vi "Read Timestamp Configuration.vi"(8 "error in (no error)":errorcluster, 9 "Default If Not Found":timestamp, 10 "Name":string, 11 "database-configuration in":refnum<class "configuration-database.lvclass">) -> (0 "error out":errorcluster, 1 "Not Found?":bool, 2 "Value":timestamp, 3 "database-configuration out":refnum<class "configuration-database.lvclass">)   [LabVIEW 2020, in "configuration-database.lvlib" / "configuration-database.lvclass"]
uses:
  configuration-database.lvclass
  configuration-database.lvclass/configuration-database.ctl
  bcf94244-2e74-4bc5-bce3-b07433e8a1bf.vi
  <vilib>/Utility/error.llb/Error Cluster From Error Code.vi
  IConfigDBQueries/IConfigurationDatabaseQueries.lvclass
  externals/database-interface/IDatabase/IDatabase/IDatabase.lvclass
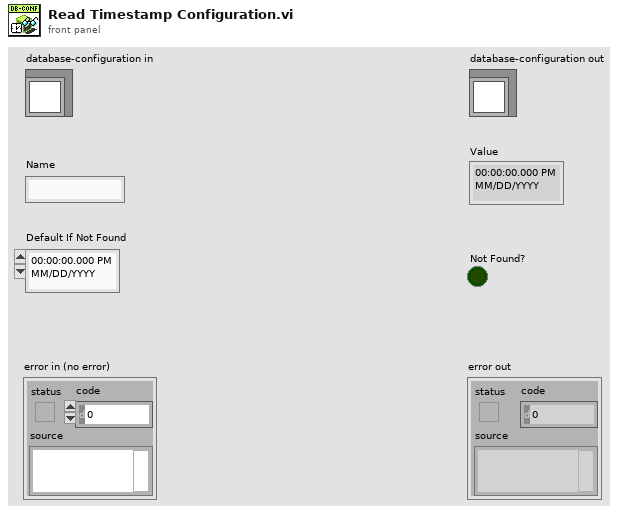
[diagram p1: front panel]
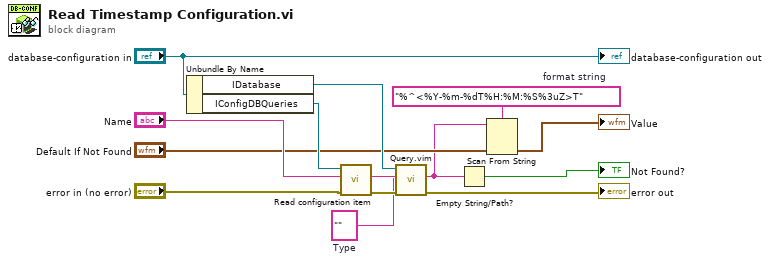
[diagram p0: block diagram]
diagram:
  w1 = ""  # Type
  w2 = "%^<%Y-%m-%dT%H:%M:%S%3uZ>T"  # format string
  n1 = Unbundle By Name("database-configuration in") -> ("IDatabase"=w13:refnum<class "IDatabase.lvclass">, "IConfigDBQueries"=w14:refnum<class "IConfigurationDatabaseQueries.lvclass">)
  n2 = call-dynamic "Read configuration item.vi"("error in (no error)"="error in (no error)", "configuration item"="Name", "IConfigDBQueries in"=w14) -> ("error out"=w12:errorcluster, "result"=w11:string)  [unwired: 7 in]
  n3 = call "Query.vim"("error in (no error)"=w12, "Type and Default"=w1, "Query string"=w11, "IDatabase in"=w13) -> ("error out"=→"error out":errorcluster, "Result"=w5:string)  [unwired: 5 in, 1 out]
  n4 = Empty String/Path?(string/path=w5) -> (empty?=→"Not Found?":bool)
  n5 = Scan From String(format string=w2, input string=w5, default 1="Default If Not Found") -> (output 1=→"Value":timestamp)  [unwired: 2 in, 3 out]
  "database-configuration out" <- "database-configuration in"
